vi "helper-points to image.vi"(11 "Array of Points":cluster{"X":dbl, "Y":dbl}[](array[cluster])) -> (3 "Image Out":T1)   [LabVIEW 2011]
doc: "Takes a list of x/y points between -10 and 10, originally meant for a plot, and overlays them on an image instead.\nPurpose: to allow for the same indicator to be used for the camera as for the simulation.\n\nBy: Jason"
uses:
  <vilib>/vision/Image Controls.llb/IMAQ Image.ctl
panel:
  out "x+y":cluster{"X":i32, "Y":i32}[](array[cluster])
  out "Image":T1(plugin-control)
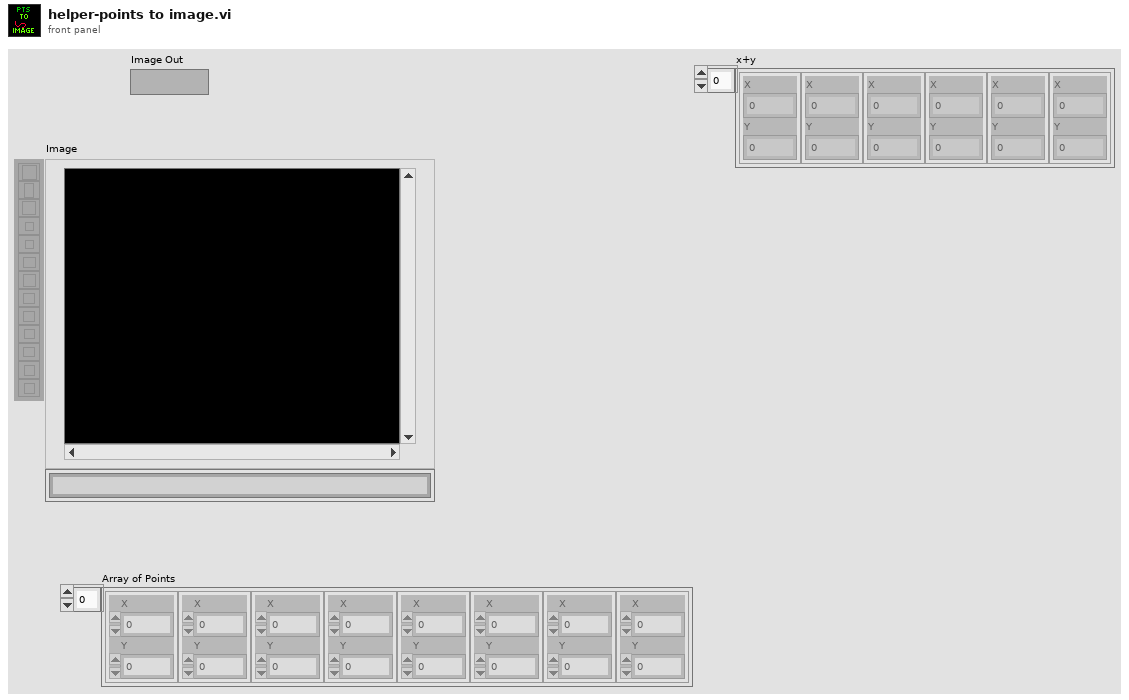
[diagram p1: front panel]
types:
  T1 = typedef "IMAQ Image.ctl" = refnum<image>
  T2 = typedef "Image Type" = u32
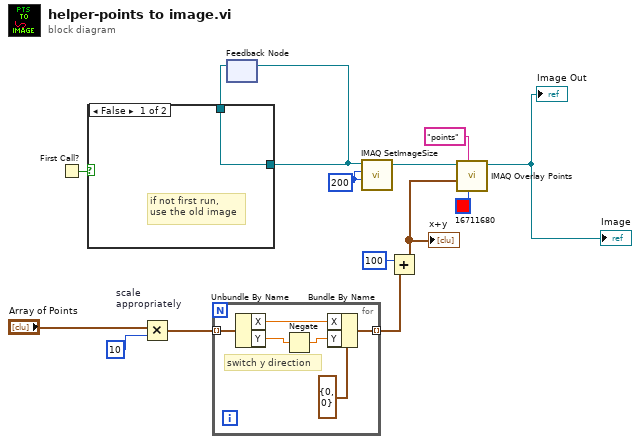
[diagram p0: block diagram]
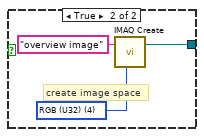
[diagram p2: hidden frame]
diagram:
  w9 = 200 ("X Resolution")
  n1 = First Call?() -> (First Call?: T/F=w14:bool)
  n2 = Multiply "scale\nappropriately"(x="Array of Points", y=10) -> (x*y=w4:cluster{"X":dbl, "Y":dbl}[])
  n3 = for {
    tunnel: w4 -> [w20] mode=indexing
    tunnel: [w19] -> w3 mode=indexing
    # "switch y direction"
    n4 = Unbundle By Name(w20) -> ("X"=w18:dbl, "Y"=w17:dbl)
    n5 = Negate(x=w17) -> (-x=w16:dbl)
    n6 = Bundle By Name(cluster=cluster{"X":i32, "Y":i32} {"X"=0, "Y"=0} ("Point Coordinates"), "X"=w18, "Y"=w16) -> (w19:cluster{"X":i32, "Y":i32})
  }
  n7 = feedback #1() -> (w12:T1)  [unwired: 1 in]
  n8 = case shown="False" w14 {
    tunnel: [w21 w23] -> w10
    tunnel: w12 -> [w21 _]
    frame False {
      # "if not first run,\nuse the old image"
    }
    frame True {
      w22 = T2 4 items=["Grayscale (U8)", "Grayscale (I16)", "Grayscale (SGL)", "Complex (CSG)", "RGB (U32)", "HSL (U32)", "RGB (U64)", "Grayscale (U16)"] ("Image Type")
      # "create image space"
      n9 = call "IMAQ Create"("Image Name"="overview image", "Image Type"=w22) -> ("New Image"=w23:T1)  [unwired: 3 in, 1 out]
    }
  }
  n10 = feedback-in #1(w10) -> ()
  n11 = call "IMAQ SetImageSize"("Y Resolution"=w9, "X Resolution"=w9, "Image"=w10) -> ("Image Out"=w11:T1)  [unwired: 2 in, 1 out]
  n12 = Add(x=100, y=w3) -> (x+y=w8:cluster{"X":i32, "Y":i32}[])
  "x+y" <- w8
  n13 = call "IMAQ Overlay Points"("Color"=u32 16711680, "Group"="points" ("points"), "Array of Points"=w8, "Image"=w11) -> ("Image Out"=→"Image Out" →"Image":T1)  [unwired: 6 in, 1 out]
